vi "Configure Session.vi"(8 "error in":errorcluster, 11 "Plugin in":refnum<class "Digital Output Handler.lvclass">) -> (0 "error out":errorcluster, 3 "Plugin out":refnum<class "Digital Output Handler.lvclass">)   [LabVIEW 2023, in "Digital Output Handler.lvlib" / "Digital Output Handler.lvclass"]
uses:
  Digital Output Handler.lvclass
  Digital Output Handler.lvclass/Digital Output Handler.ctl
  <vilib>/FlexLogger/SDK/PluginSDK.lvlibp/PEFClasses/SDK/Channel/Data Type_v2.ctl
  <vilib>/FlexLogger/SDK/PluginSDK.lvlibp/PEFClasses/SDK/Setpoint Consumer Channel/Setpoint Consumer Channel.lvclass
  <vilib>/FlexLogger/SDK/PluginSDK.lvlibp/PEFClasses/SDK/Producer Channel/Producer Channel.lvclass
  <vilib>/FlexLogger/SDK/PluginSDK.lvlibp/PEFClasses/SDK/Plugin/ParameterAccess/Read I32.vi
  <vilib>/FlexLogger/SDK/PluginSDK.lvlibp/PEFClasses/SDK/Derived Timing Producer Channel/Create Derived Time Producer Channel_v2.vi
  <vilib>/FlexLogger/SDK/PluginSDK.lvlibp/PEFClasses/SDK/Setpoint Consumer Channel/Create Setpoint Consumer Channel.vi
  <vilib>/FlexLogger/SDK/PluginSDK.lvlibp/PEFClasses/SDK/Channel/Channel.lvclass
  <vilib>/FlexLogger/SDK/PluginSDK.lvlibp
  <vilib>/FlexLogger/SDK/PluginSDK.lvlibp/PEFClasses/SDK/Plugin/Plugin.lvclass
  <vilib>/FlexLogger/SDK/PluginSDK.lvlibp/PEFClasses/SDK/Derived Timing Producer Channel/Derived Timing Producer Channel.lvclass
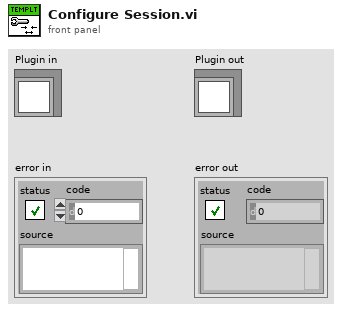
[diagram p1: front panel]
types:
  T1 = typedef "PluginSDK.lvlibp/Channel.lvclass/Data Type_v2.ctl" = u16
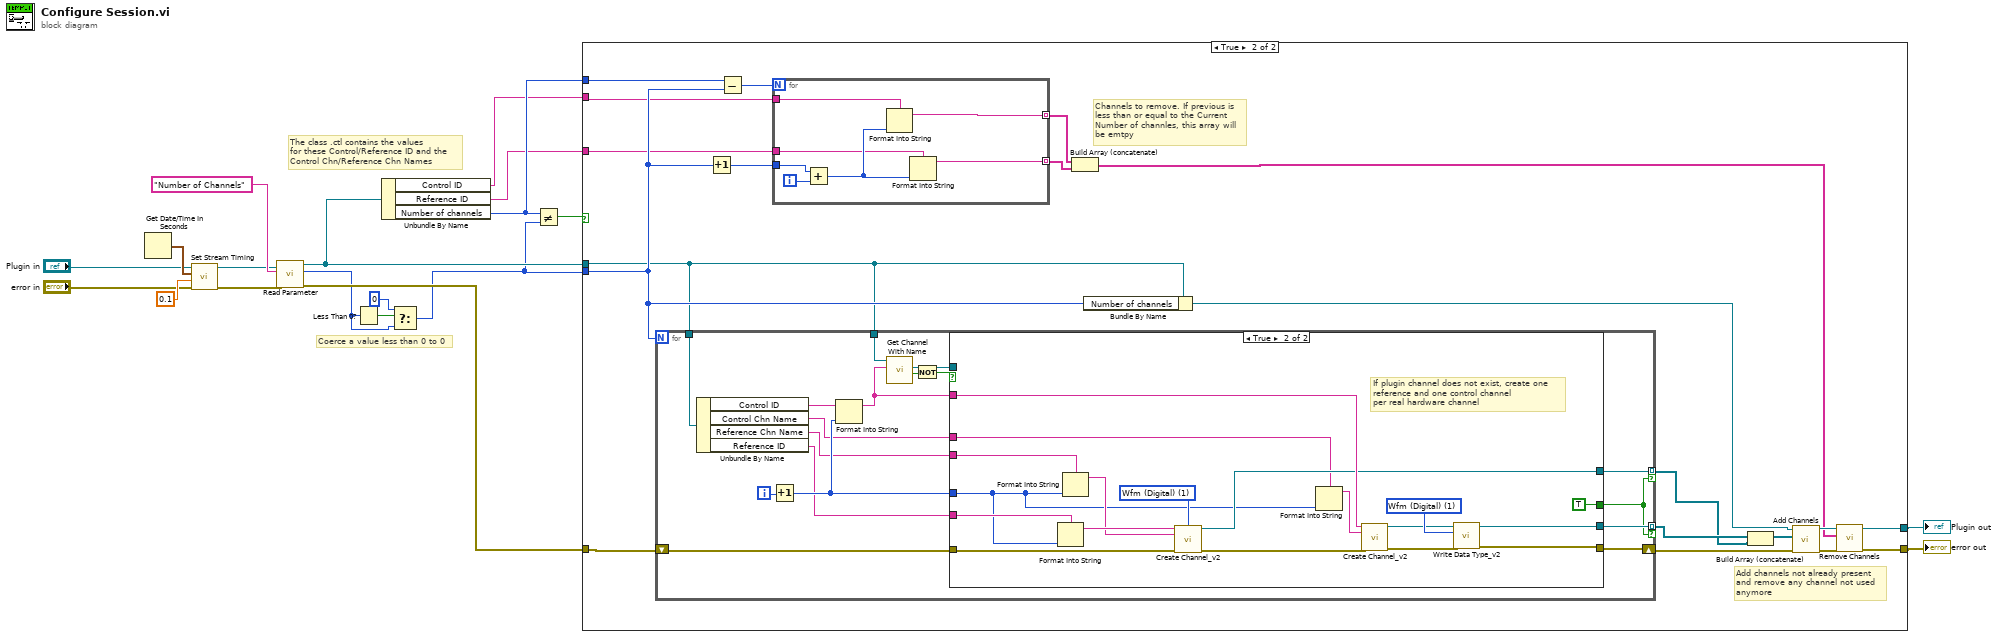
[diagram p0: block diagram]
diagram:
  # "Coerce a value less than 0 to 0"
  # "The class .ctl contains the values\nfor these Control/Reference ID and the\nControl Chn/Reference Chn Names"
  n1 = Get Date/Time In Seconds() -> (seconds since 1Jan1904=w9:timestamp)
  n2 = call-dynamic "Set Stream Timing.vi"("error in (no error)"="error in", "dt(sec)"=0.1, "Start Time"=w9, "Plugin in"="Plugin in") -> ("error out"=w7:errorcluster, "Plugin out"=w6:refnum<class "Digital Output Handler.lvclass">)  [unwired: 6 in]
  n3 = call-poly <vilib>:"Read Parameter.vi"("error in (no error)"=w7, "Name"="Number of Channels", "Plugin in"=w6) -> ("error out"=w17:errorcluster, "Value"=w2:i32, "Plugin out"=w14:refnum<class "Digital Output Handler.lvclass">)  [unwired: 5 in, 1 out]
  n4 = Less Than 0?(x=w2) -> (x < 0?=w4:bool)
  n5 = Unbundle By Name(w14) -> ("Control ID"=w12:string, "Reference ID"=w11:string, "Number of channels"=w13:i32)
  n6 = Select(t=0, s=w4, f=w2) -> (s? t:f=w3:i32)
  n7 = Not Equal?(x=w13, y=w3) -> (x != y?=w18:bool)
  n8 = case shown="True" w18 {
    tunnel: w17 -> [w20 w41]
    tunnel: w14 -> [w21 w22]
    tunnel: w13 -> [_ w27]
    tunnel: w3 -> [_ w25]
    tunnel: [w21 w35] -> w16
    tunnel: [w20 w34] -> w15
    tunnel: w12 -> [_ w24]
    tunnel: w11 -> [_ w23]
    frame False {
    }
    frame True {
      # "Add channels not already present\nand remove any channel not used\nanymore"
      # "Channels to remove. If previous is less than or equal to the Current Number of channles, this array will be emtpy"
      n9 = for {
        N: w25 -> [_]
        tunnel: w22 -> [w58]
        tunnel: [w53] -> w37 mode=indexing if=w51
        tunnel: [w52] -> w38 mode=indexing if=w51
        shift-right: [w54] -> w36
        shift-left: w41 -> [w55]
        tunnel: w22 -> [w46]
        i -> [w50]
        n10 = Unbundle By Name(w46) -> ("Control ID"=w45:string, "Control Chn Name"=w43:string, "Reference Chn Name"=w44:string, "Reference ID"=w42:string)
        n11 = Increment(x=w50) -> (x+1=w48:i32)
        n12 = Format Into String(format string=w45, w48) -> (resulting string=w47:string)  [unwired: 2 in, 1 out]
        n13 = call <vilib>:"Get Channel With Name.vi"("Name"=w47, "Plugin in"=w58) -> ("Found?"=w57:bool, "Channel"=w49:refnum<class "Channel.lvclass">)  [unwired: 7 in, 1 out]
        n14 = Not(x=w57) -> (.not. x?=w56:bool)
        n15 = case shown="True" w56 {
          tunnel: w55 -> [w59 w75]
          tunnel: [_ w66] -> w52
          tunnel: [_ w69] -> w53
          tunnel: [w59 w67] -> w54
          tunnel: [_ TRUE] -> w51
          tunnel: w49 -> [_ _]
          tunnel: w48 -> [_ w60]
          tunnel: w47 -> [_ w71]
          tunnel: w44 -> [_ w63]
          tunnel: w43 -> [_ w62]
          tunnel: w42 -> [_ w61]
          frame False {
            # "If plugin channel is already present do nothing"
          }
          frame True {
            w68 = T1 1 items=["Wfm (DBL)", "Wfm (Digital)", "String"] ("Data Type")
            w76 = T1 1 items=["Wfm (DBL)", "Wfm (Digital)", "String"] ("Data Type")
            # "If plugin channel does not exist, create one\nreference and one control channel\nper real hardware channel"
            n16 = Format Into String(format string=w61, w60) -> (resulting string=w77:string)  [unwired: 2 in, 1 out]
            n17 = Format Into String(format string=w63, w60) -> (resulting string=w72:string)  [unwired: 2 in, 1 out]
            n18 = call-poly <vilib>:"Create Channel_v2.vi"("Unique Channel Identifier"=w77, "Data Type"=w76, "Default Channel Name"=w72, "error in (no error)"=w75) -> ("Producer Channel"=w69:refnum<class "Producer Channel.lvclass">, "error out"=w70:errorcluster)  [unwired: 10 in]
            n19 = Format Into String(format string=w62, w60) -> (resulting string=w73:string)  [unwired: 2 in, 1 out]
            n20 = call-poly <vilib>:"Create Channel_v2.vi"("Unique Channel Identifier"=w71, "Default Channel Name"=w73, "error in (no error)"=w70) -> ("Setpoint Consumer Channel"=w64:refnum<class "Setpoint Consumer Channel.lvclass">, "error out"=w65:errorcluster)  [unwired: 11 in]
            n21 = call-dynamic "Write Data Type_v2.vi"("error in (no error)"=w65, "Data Type"=w68, "Channel in"=w64) -> ("error out"=w67:errorcluster, "Channel out"=w66:refnum<class "Setpoint Consumer Channel.lvclass">)  [unwired: 7 in]
          }
        }
      }
      n22 = Increment(x=w25) -> (x+1=w26:i32)
      n23 = Subtract(x=w27, y=w25) -> (x-y=w28:i32)
      n24 = for {
        N: w28 -> [_]
        tunnel: [w84] -> w40 mode=indexing
        tunnel: [w83] -> w39 mode=indexing
        tunnel: w26 -> [w80]
        tunnel: w24 -> [w79]
        tunnel: w23 -> [w78]
        i -> [w82]
        n25 = Add(x=w80, y=w82) -> (x+y=w81:i32)
        n26 = Format Into String(format string=w79, w81) -> (resulting string=w84:string)  [unwired: 2 in, 1 out]
        n27 = Format Into String(format string=w78, w81) -> (resulting string=w83:string)  [unwired: 2 in, 1 out]
      }
      n28 = Build Array (concatenate)(w40, w39) -> (w29:string[])
      n29 = Bundle By Name(cluster=w22, "Number of channels"=w25) -> (w31:refnum<class "Digital Output Handler.lvclass">)
      n30 = Build Array (concatenate)(w38, w37) -> (w30:refnum<class "Channel.lvclass">[])
      n31 = call <vilib>:"Add Channels.vi"("error in (no error)"=w36, "Channels"=w30, "Plugin in"=w31) -> ("error out"=w33:errorcluster, "Plugin out"=w32:refnum<class "Digital Output Handler.lvclass">)  [unwired: 7 in]
      n32 = call-dynamic "Remove Channels.vi"("error in (no error)"=w33, "Unique Channel Identifiers to Delete"=w29, "Plugin in"=w32) -> ("error out"=w34:errorcluster, "Plugin out"=w35:refnum<class "Digital Output Handler.lvclass">)  [unwired: 7 in]
    }
  }
  "error out" <- w15
  "Plugin out" <- w16
